vi "XIPIN_Aurora_64B66B_11_0.vi"   [LabVIEW 2017]
doc: "This is Aurora 64B66B V11.0 core.Customizable multi-lane gigabit serial link implementing the Aurora 64B/66B protocol\n------------------------------------\n<b>Need License</b> : No\n<b>Interface</b> : AXI4 AXI4-Stream"
uses:
  <vilib>/rvi/XilinxIP/XIPIN_XNode/niFpgaXIPIN.xnode
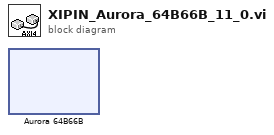
[diagram p0: block diagram]
diagram:
  n1 = xnode ("Aurora 64B66B")() -> ()
